vi "Autonomous.vi"   [LabVIEW 2015]
doc: "This VI starts when autonomous period begins, and will automatically be terminated when it ends. You can carry out timed or sensor driven operations directly to I/O or to subsystems without needing to return to the caller."
uses:
  <vilib>/Rock Robotics/Network Tables/NT Read String.vi
types:
  T1 = typedef "WPI_JoystickDevRef.ctl" = cluster{"Device":T2}
  T2 = typedef "WPI_JoystickDeviceEnum.ctl" = enum16{"USB 0", "USB 1", "USB 2", "USB 3", "USB 4", "USB 5"}
  T3 = typedef "WPI_RobotDriveDevRef.ctl" = cluster{"DevStatus":errorcluster, "Motors[]":T4[], "Square Inputs":bool, "Max Output":dbl}
  T4 = typedef "WPI_MotorControlDeviceRef.ctl" = cluster{"DeviceStatus":errorcluster, "Type":T5, "PWM":cluster{"PWM Channel":T6, "DeadBand":T7}, "CAN":cluster{"Device Number":u8, "Control Mode":T8, "Semaphore":T9, "Max Vout":dbl, "TalonSRX Control Mode":T10}, "Invert":bool}
  T5 = typedef "WPI_MotorControlType.ctl" = enum16{"PWM", "CAN", "CANTalonSRX"}
  T6 = typedef "FPGA_DIOPWMChannel.ctl" = enum8{"PWM 0", "PWM 1", "PWM 2", "PWM 3", "PWM 4", "PWM 5", "PWM 6", "PWM 7", "PWM 8", "PWM 9", "PWM MXP 0", "PWM MXP 1", "PWM MXP 2", "PWM MXP 3", "PWM MXP 4", "PWM MXP 5", "PWM MXP 6", "PWM MXP 7", "PWM MXP 8", "PWM MXP 9", "Invalid"}
  T7 = typedef "WPI_PWMDeadband.ctl" = cluster{"Name":string, "maxPositivePwm":i32, "minPositivePwm":i32, "centerPwm":i32, "maxNegativePwm":i32, "minNegativePwm":i32, "angularRange":u16}
  T8 = typedef "WPI_CANJaguar_ControlMode.ctl" = enum8{"Percent VBus", "Current", "Speed", "Position", "Voltage"}
  T9 = typedef "Semaphore RefNum" = refnum<k1>
  T10 = typedef "WPI_CANTalonSRX_APIControlMode.ctl" = enum8{"Percent VBus", "Speed", "Position", "Slave", "Unchanged / Invalid", "Voltage Compensation", "Current", "Motion Profile"}
  T11 = typedef "Command Status Info.ctl" = cluster{"Name":string, "Status":T12, "notifier out":T13}
  T12 = typedef "Completion Status.ctl" = enum16{"Successful", "Aborted", "Incomplete"}
  T13 = typedef "Completion Notifier.ctl" = refnum<notifier>
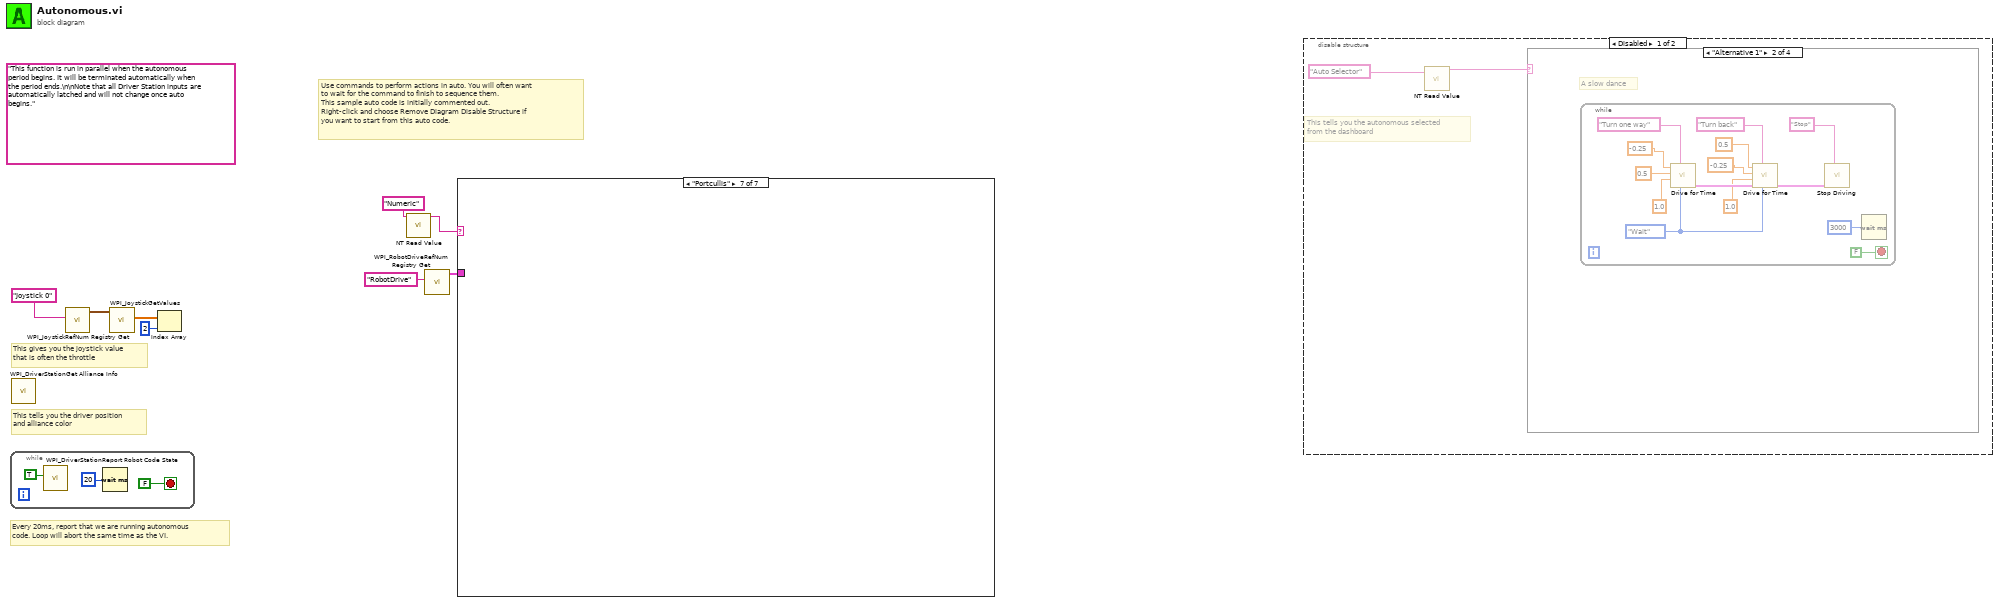
[diagram p0: block diagram]
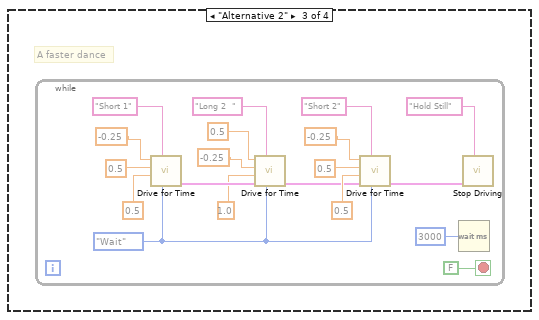
[diagram p9: hidden frame]
diagram:
  (unwired) "This function is run in parallel when the autonomous period begins. It will be terminated automatically when the period ends.\n\nNote that all Driver Station inputs are automatically latched and will not change once auto begins."
  # "Every 20ms, report that we are running autonomous\ncode. Loop will abort the same time as the VI."
  # "This gives you the joystick value\nthat is often the throttle"
  # "Use commands to perform actions in auto. You will often want\nto wait for the command to finish to sequence them.\nThis sample auto code is initially commented out. \nRight-click and choose Remove Diagram Disable Structure if\nyou want to start from this auto code."
  # "This tells you the driver position\nand alliance color"
  n1 = while {
    stop <- FALSE stop-if-true
    n2 = call <vilib>:"WPI_DriverStationReport Robot Code State.vi"("Autonomous"=TRUE) -> ()  [unwired: 10 in, 1 out]
    n3 = Wait (ms)(milliseconds to wait=u32 20) -> ()  [unwired: 1 out]
  }
  n4 = call <vilib>:"WPI_DriverStationGet Alliance Info.vi"() -> ()  [unwired: 12 out]
  n5 = call <vilib>:"WPI_JoystickRefNum Registry Get.vi"("refnum name"="Joystick 0") -> ("JoystickDevRef"=w7:T1)  [unwired: 1 in, 9 out]
  n6 = call <vilib>:"WPI_JoystickGetValues.vi"("JoystickDevRef"=w7) -> ("Axes"=w6:dbl[])  [unwired: 6 in, 4 out]
  n7 = Index Array(array=w6, index=2) -> ()  [unwired: 1 out]
  n8 = call-poly <vilib>:"NT Read Value.vi"("Name"="Numeric") -> ("String"=w3:string)  [unwired: 9 in, 1 out]
  n9 = call <vilib>:"WPI_RobotDriveRefNum Registry Get.vi"("refnum name"="RobotDrive") -> ("RobotDriveDevRef"=w1:T3)  [unwired: 9 in, 1 out]
  n10 = case shown="\"Portcullis\"" w3 {
    tunnel: w1 -> [_ _ _ _ _ _ _]
    frame "Cheval de Frise" {
    }
    frame "Moat" {
    }
    frame "Ramparts" {
    }
    frame "Rockwall" {
    }
    frame "Rough Terrain" {
    }
    frame "Low Bar" {
    }
    frame "Portcullis" {
    }
  }
  n11 = disable-structure shown="Disabled" {
    frame Disabled {
      # "This tells you the autonomous selected\nfrom the dashboard"
      n12 = call-poly <vilib>:"NT Read Value.vi"("Name"="Auto Selector") -> ("String"=w12:string)  [unwired: 9 in, 1 out]
      n13 = case shown="\"Alternative 1\"" w12 {
        frame Default {
          # "You can put your main auto here, or you can right-click on the case and make any\nother frame be the default case."
          # "This is the frame that will execute if no selection is made, or if it is not recognized"
        }
        frame "Alternative 1" {
          # "A slow dance"
          n14 = while {
            stop <- FALSE stop-if-true
            w18 = enum16{"Start", "Wait"}."Wait" ("Synchronication")
            n15 = call "Drive for Time.vi"("Synchronization"=w18, "Description"="Turn one way", "Seconds"=1.0 ("Delay (s)"), "Right Speed"=0.5 ("X axis value"), "Left Speed"=-0.25 ("X axis value")) -> ("Command Info Out"=w27:T11)  [unwired: 5 in, 1 out]
            n16 = call "Drive for Time.vi"("Synchronization"=w18, "Description"="Turn back", "Command Info In"=w27, "Seconds"=1.0 ("Delay (s)"), "Right Speed"=-0.25 ("X axis value"), "Left Speed"=0.5 ("X axis value")) -> ("Command Info Out"=w17:T11)  [unwired: 4 in, 1 out]
            n17 = call "Stop Driving.vi"("Description"="Stop", "Command Info In"=w17) -> ()  [unwired: 9 in, 1 out]
            n18 = Wait (ms)(milliseconds to wait=u32 3000 ("millisecond timer value")) -> ()  [unwired: 1 out]
          }
        }
        frame "Alternative 2" {
          # "A faster dance"
          n19 = while {
            stop <- FALSE stop-if-true
            w28 = enum16{"Start", "Wait"}."Wait" ("Synchronication")
            n20 = call "Drive for Time.vi"("Synchronization"=w28, "Description"="Short 1", "Seconds"=0.5 ("Delay (s)"), "Right Speed"=0.5 ("X axis value"), "Left Speed"=-0.25 ("X axis value")) -> ("Command Info Out"=w46:T11)  [unwired: 5 in, 1 out]
            n21 = call "Drive for Time.vi"("Synchronization"=w28, "Description"="Long 2  ", "Command Info In"=w46, "Seconds"=1.0 ("Delay (s)"), "Right Speed"=-0.25 ("X axis value"), "Left Speed"=0.5 ("X axis value")) -> ("Command Info Out"=w30:T11)  [unwired: 4 in, 1 out]
            n22 = call "Drive for Time.vi"("Synchronization"=w28, "Description"="Short 2", "Command Info In"=w30, "Seconds"=0.5 ("Delay (s)"), "Right Speed"=0.5 ("X axis value"), "Left Speed"=-0.25 ("X axis value")) -> ("Command Info Out"=w29:T11)  [unwired: 4 in, 1 out]
            n23 = Wait (ms)(milliseconds to wait=u32 3000 ("millisecond timer value")) -> ()  [unwired: 1 out]
            n24 = call "Stop Driving.vi"("Description"="Hold Still", "Command Info In"=w29) -> ()  [unwired: 9 in, 1 out]
          }
        }
        frame "Your Turn" {
        }
      }
    }
    frame Enabled {
    }
  }
